vi "2016 Controller logging.vi"() -> ()   [LabVIEW 2015]
uses:
  <vilib>/Rock Robotics/WPI/Joystick/WPI_JoystickDeviceEnum.ctl
panel:
  out "spreadsheet string":string
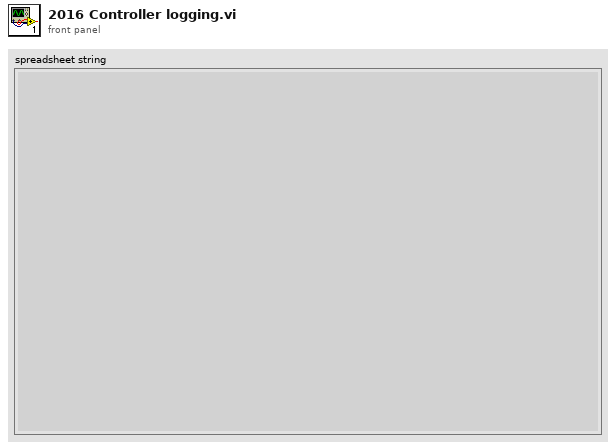
[diagram p1: front panel]
types:
  T1 = typedef "WPI_JoystickDeviceEnum.ctl" = enum16{"USB 0", "USB 1", "USB 2", "USB 3", "USB 4", "USB 5"}
  T2 = typedef "WPI_JoystickDevRef.ctl" = cluster{"Device":T1}
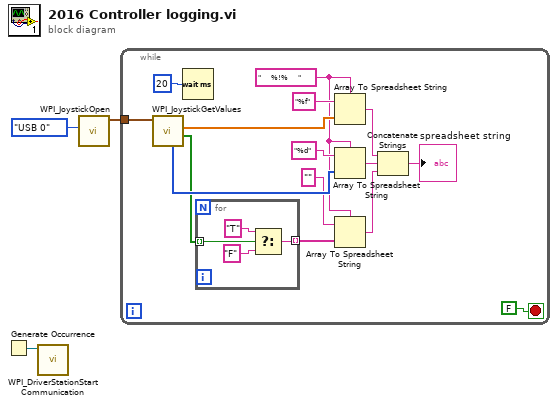
[diagram p0: block diagram]
diagram:
  n1 = Generate Occurrence() -> (w3:refnum<k4>)
  n2 = call <vilib>:"WPI_DriverStationStart Communication.vi"("occurrence"=w3) -> ()  [unwired: 11 in]
  n3 = call <vilib>:"WPI_JoystickOpen.vi"("JoystickDevice"=WPI_JoystickDeviceEnum."USB 0") -> ("JoystickDevRef"=w2:T2)  [unwired: 10 in]
  n4 = while {
    tunnel: w2 -> [w18]
    stop <- FALSE stop-if-true
    w9 = "     %!%     " ("delimiter (Tab)")
    n5 = call <vilib>:"WPI_JoystickGetValues.vi"("JoystickDevRef"=w18) -> ("Buttons"=w11:bool[], "Axes"=w13:dbl[], "POVs"=w14:i16[])  [unwired: 6 in, 2 out]
    n6 = Wait (ms)(milliseconds to wait=u32 20) -> ()  [unwired: 1 out]
    n7 = for {
      tunnel: w11 -> [w22] mode=indexing
      tunnel: [w19] -> w10 mode=indexing
      n8 = Select(t="T", s=w22, f="F") -> (s? t:f=w19:string)
    }
    n9 = Array To Spreadsheet String(delimiter (Tab)=w9, array=w13, 3:"%f" ("format string")) -> (spreadsheet string=w6:string)
    n10 = Array To Spreadsheet String(delimiter (Tab)=w9, array=w14, 3:"%d" ("format string")) -> (spreadsheet string=w5:string)
    n11 = Array To Spreadsheet String(delimiter (Tab)=w9, array=w10, 3:"" ("format string")) -> (spreadsheet string=w4:string)
    n12 = Concatenate Strings(w6, w5, w4) -> (→"spreadsheet string":string)
  }
